vi "test_4_1 (SubVI).vi"(0 "Voltage":dbl, 5 "y":i32=100, 7 "Lux":dbl format="%#_13g", 9 "Numeric":i32, 11 "Filename":path=path "C:/Users/Dyakov_AVi/Nextcloud/bioreactor_labview/test_1.lvm") -> ()   [LabVIEW 2016]
uses:
  <vilib>/express/express shared/transition.llb/Dynamic To Waveform Array.vi
  <vilib>/express/express signal manip/GetorSetDDTAttributes/Set DDT Attributes/SetT0.vi
  <vilib>/express/express shared/transition.llb/Waveform Array To Dynamic.vi
  <vilib>/express/express signal manip/GetorSetDDTAttributes/Set DDT Attributes/Set DDT Properties.xnode
  <vilib>/ptbypt/NI_PtbyPt.lvlib
panel:
  out "m":dbl
  out "s":dbl
  out "relative seconds":dbl format="%_19f"
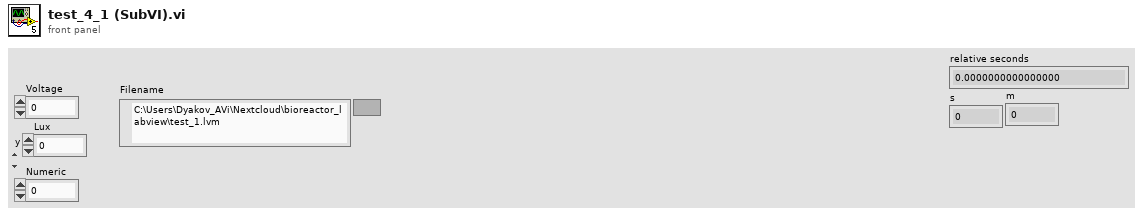
[diagram p1: front panel]
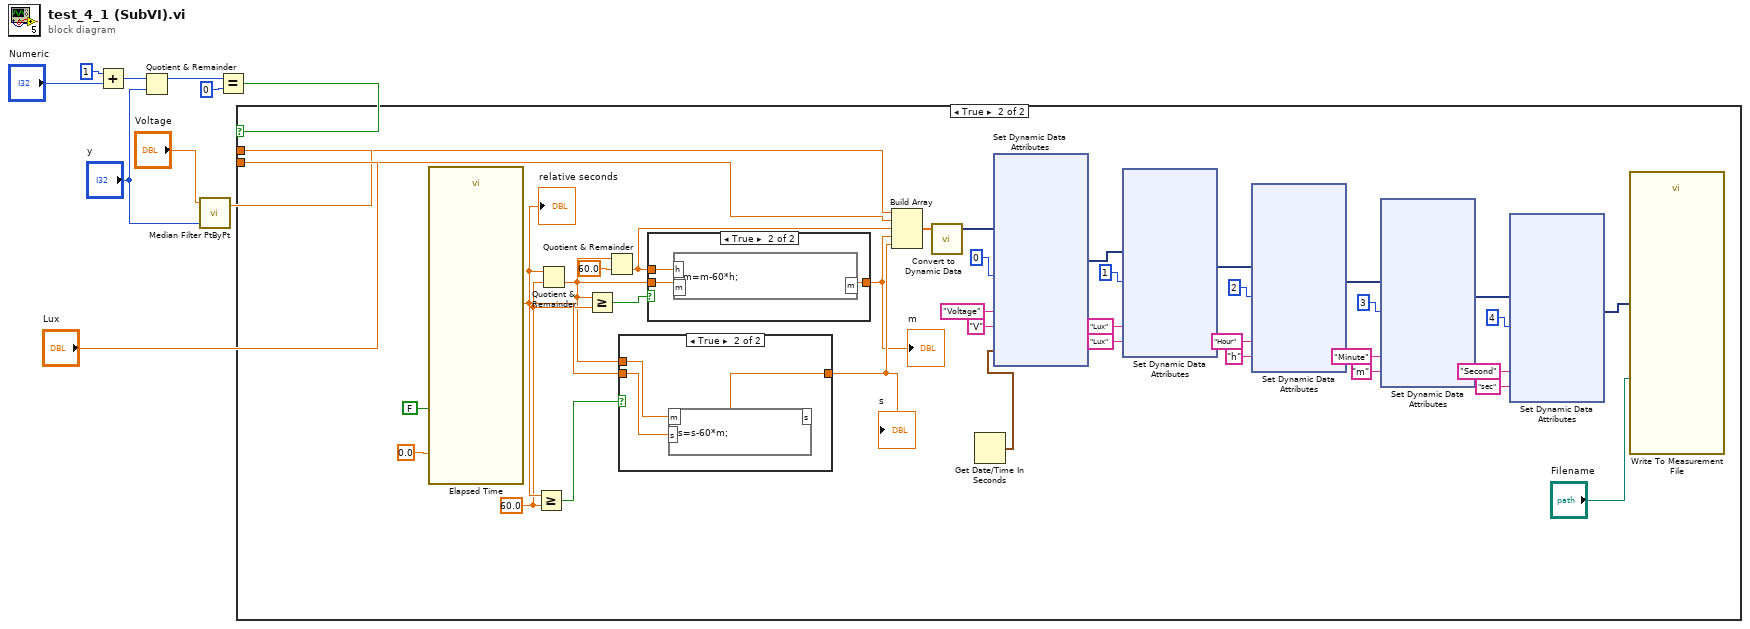
[diagram p0: block diagram]
diagram:
  n1 = Add(x=1, y="Numeric") -> (x+y=w6:i32)
  n2 = Quotient & Remainder(x=w6, y="y") -> (x-y*floor(x/y)=w3:i32)  [unwired: 1 out]
  n3 = call <vilib>:"Median Filter PtByPt.vi"("rank"="y", "x"="Voltage") -> ("Filtered x"=w1:dbl)  [unwired: 2 in, 1 out]
  n4 = Equal?(x=w3, y=0) -> (x = y?=w9:bool)
  n5 = case shown="True" w9 {
    tunnel: "Lux" -> [_ w22]
    tunnel: w1 -> [_ w46]
    frame False {
    }
    frame True {
      w27 = 60.0 ("y")
      n6 = call "Elapsed Time"("Auto Reset"=FALSE, "Set Start Time (s)"=0.0) -> ("Elapsed Time (s)"=w29:dbl)  [unwired: 10 in, 7 out]
      "relative seconds" <- w29
      n7 = Greater Or Equal?(x=w29, y=w27) -> (x >= y?=w30:bool)
      n8 = Quotient & Remainder(x=w29, y=w27) -> (floor(x/y)=w23:dbl)  [unwired: 1 out]
      n9 = Greater Or Equal?(x=w23, y=w27) -> (x >= y?=w26:bool)
      n10 = Quotient & Remainder(x=w23, y=60.0) -> (floor(x/y)=w25:dbl)  [unwired: 1 out]
      n11 = case shown="True" w30 {
        tunnel: w29 -> [w52 w55]
        tunnel: w23 -> [_ w54]
        tunnel: [w52 w53] -> w28
        frame False {
        }
        frame True {
          n12 = formula code="s=s-60*m;"("s"=w55, "m"=w54) -> ("s"=w53:dbl)
        }
      }
      "s" <- w28
      n13 = case shown="True" w26 {
        tunnel: w23 -> [w48 w51]
        tunnel: w25 -> [_ w50]
        tunnel: [w48 w49] -> w24
        frame False {
        }
        frame True {
          n14 = formula code="m=m-60*h;"("m"=w51, "h"=w50) -> ("m"=w49:dbl)
        }
      }
      "m" <- w24
      n15 = Build Array(w46, w22, w25, w24, w28) -> (w45:dbl[])
      n16 = call "Convert to Dynamic Data"("Array"=w45) -> ("Dynamic Data Type"=w32:dynamicdata)  [unwired: 3 in]
      n17 = Get Date/Time In Seconds() -> (seconds since 1Jan1904=w11:timestamp)
      n18 = xnode "Set Dynamic Data Attributes"("Signals In"=w32, "Signal Index"=0, "Signal Name"="Voltage", "Unit"="V", "Timestamp"=w11) -> ("Signals Out"=w44:dynamicdata)  [unwired: 1 in, 1 out]
      n19 = xnode "Set Dynamic Data Attributes"("Signals In"=w44, "Signal Index"=1, "Signal Name"="Lux", "Unit"="Lux") -> ("Signals Out"=w39:dynamicdata)  [unwired: 1 in, 1 out]
      n20 = xnode "Set Dynamic Data Attributes"("Signals In"=w39, "Signal Index"=2, "Signal Name"="Hour", "Unit"="h") -> ("Signals Out"=w38:dynamicdata)  [unwired: 1 in, 1 out]
      n21 = xnode "Set Dynamic Data Attributes"("Signals In"=w38, "Signal Index"=3, "Signal Name"="Minute", "Unit"="m") -> ("Signals Out"=w37:dynamicdata)  [unwired: 1 in, 1 out]
      n22 = xnode "Set Dynamic Data Attributes"("Signals In"=w37, "Signal Index"=4, "Signal Name"="Second", "Unit"="sec") -> ("Signals Out"=w36:dynamicdata)  [unwired: 1 in, 1 out]
      n23 = call "Write To Measurement File"("Signals"=w36, "Filename"="Filename") -> ()  [unwired: 15 in, 3 out]
    }
  }
